vi "Tool RS232 test01.vi"(8 "error in (no error)":errorcluster, 10 "select step":T1=enum."Initial", 11 "VISA resource name":refnum<visa-resource-name>="COM3") -> (0 "error out":errorcluster)   [LabVIEW 2019]
uses:
  Ctrl/ProjectStepSelect.ctl
  Ctrl/ProjectCmdStep.ctl
  Global/Process Global.vi
panel:
  out ".not. x?":bool
  out "concatenated string":string
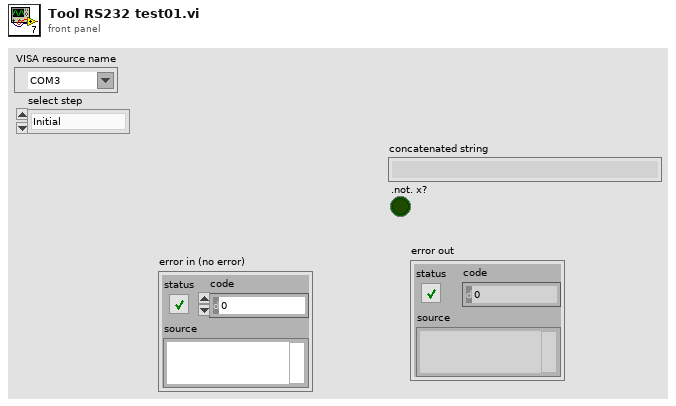
[diagram p1: front panel]
types:
  T1 = typedef "ProjectStepSelect.ctl" = enum16{"ProjectName", "Name", "Initial", "Reset", "Format", "Program1", "Program2", "Scan", "Finish", "MToolWork", "DataCheck", "DataSave", "OutputPLC", "WaitInputS1", "WaitInputOff"}
  T2 = typedef "ProjectCmdStep.ctl" = enum16{"Project Name", "commamd1", "commamd2", "commamd3", "wat time1", "return1", "return2", "return3", "wat time2", "over time", "retry"}
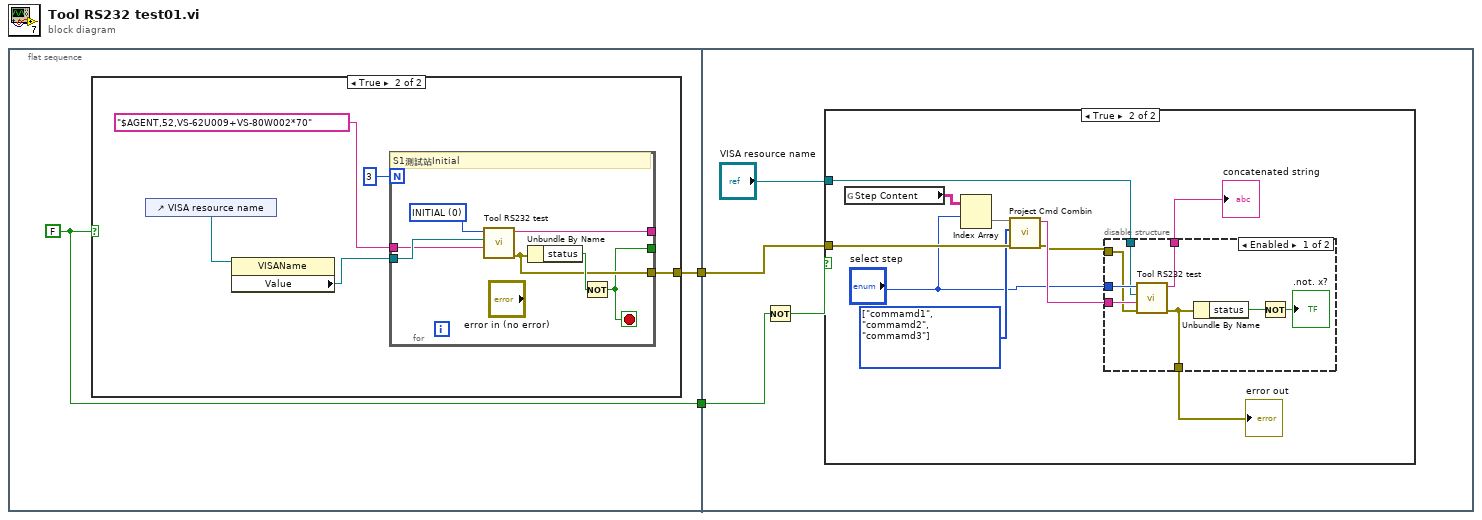
[diagram p0: block diagram]
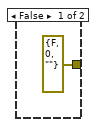
[diagram p2: hidden frame]
diagram:
  n1 = flat-sequence {
    tunnel: [w4] -> w2
    tunnel: [w3] -> w1
    tunnel: w2 -> [w21]
    tunnel: w1 -> [w20]
    frame #0 {
      w3 = FALSE
      n2 = case shown="True" w3 {
        tunnel: [errorcluster {"status"=FALSE, "code"=0, "source"=""} ("error out") w10] -> w4
        frame False {
        }
        frame True {
          n3 = control-ref of="VISA resource name"() -> (w7:refnum<vi>)
          n4 = property class="VISAName"(reference=w7) -> ("Value"=w6:refnum<visa-resource-name>)  [unwired: 1 in, 2 out]
          n5 = for {
            N: 3 -> [_]
            tunnel: [w15] -> _
            tunnel: [w14] -> w10
            tunnel: [w13] -> _
            tunnel: w6 -> [w12]
            tunnel: "$AGENT,52,VS-62U009+VS-80W002*70" ("Cmd 2") -> [w11]
            stop <- w13 stop-if-true
            w16 = u16 0 items=["INITIAL", "RESET", "FORMAT", "PROGRAM1", "PROGRAM2", "FSKSCAN", "ASKSCAN"] ("action")
            # "S1測試站Initial"
            n6 = call "Tool RS232 test.vi"("Cmd In"=w11, "VISA resource name"=w12, "action"=w16) -> ("error out"=w14:errorcluster, "receive string"=w15:string)  [unwired: 7 in]
            n7 = Unbundle By Name(w14) -> ("status"=w17:bool)
            n8 = Not(x=w17) -> (.not. x?=w13:bool)
          }
        }
      }
    }
    frame #1 {
      n9 = Not(x=w20) -> (.not. x?=w19:bool)
      n10 = case shown="True" w19 {
        tunnel: w21 -> [_ w31]
        tunnel: "VISA resource name" -> [_ w25]
        frame False {
        }
        frame True {
          w24 = T2[] [enum."commamd1", enum."commamd2", enum."commamd3"] items=["Project Name", "commamd1", "commamd2", "commamd3", "wat time1", "return1", "return2", "return3", "wat time2", "over time", "retry"] ("Cmd Step")
          n11 = global read "Process Global.vi" "Step Content"() -> (w29:string[][])
          n12 = Index Array(array=w29, index (row)="select step") -> (element=w28:string[])  [unwired: 1 in]
          n13 = call "Project Cmd Combin.vi"("error in (no error)"=w31, "Cmd Step"=w24, "Content Input"=w28) -> ("error out"=w27:errorcluster, "concatenated string"=w30:string)  [unwired: 6 in, 1 out]
          n14 = disable-structure shown="Enabled" {
            disable-tunnel: w30 -> [w39 _]
            disable-tunnel: "select step" -> [w37 _]
            disable-tunnel: w27 -> [w36 _]
            disable-tunnel: [w34 _] -> w26
            disable-tunnel: w25 -> [w33 _]
            disable-tunnel: [w32 _] -> w22
            frame Enabled {
              n15 = call "Tool RS232 test.vi"("error in (no error)"=w36, "Cmd In"=w39, "VISA resource name"=w33, "action"=w37) -> ("error out"=w32:errorcluster, "receive string"=w34:string)  [unwired: 6 in]
              n16 = Unbundle By Name(w32) -> ("status"=w38:bool)
              n17 = Not(x=w38) -> (.not. x?=→".not. x?":bool)
            }
            frame Disabled {
            }
          }
          "concatenated string" <- w26
          "error out" <- w22
        }
      }
    }
  }
